vi "Estimator.vi"(0 "target_covariance":dbl[][](array[numeric]), 5 "nontarget_covariance":dbl[][](array[numeric]), 7 "u(t=1, 2, ...6)_target":dbl[][](array[numeric]), 9 "u(t=1, 2, ...6)_nontarget":dbl[][](array[numeric]), 11 "alk":dbl[][](array[numeric])) -> (4 "L_k(t)":ext[][](array[numeric]), 6 "H_lk":ext[][][](array[numeric]))   [LabVIEW 2013]
uses:
  <vilib>/Analysis/baseanly.llb/Real A x B.vi
  <vilib>/Analysis/Matrix/Numeric/Conversions/Array To Matrix - RA.vi
  <vilib>/Analysis/Matrix/Numeric/Conversions/Matrix To Array - RM.vi
  <vilib>/Analysis/Matrix/NI_Matrix.lvlib
  <vilib>/Analysis/NI_AALBase.lvlib
panel:
  in  "Tab Control":enum32{"ALPHA", "BETA", "L_K, H_KL"}(tab)
  out "pi":dbl[](array[numeric])
  out "u(1)_target":dbl[](array[numeric])
  out "u(1)_nontarget":dbl[](array[numeric])
  out "alpha_k(t)":ext[][](array[numeric])
  out "beta(t)":ext[][](array[numeric])
  out "P(u)":ext
  # "INPUT"
  # "INITIALIZATION"
  # "OUTPUT"
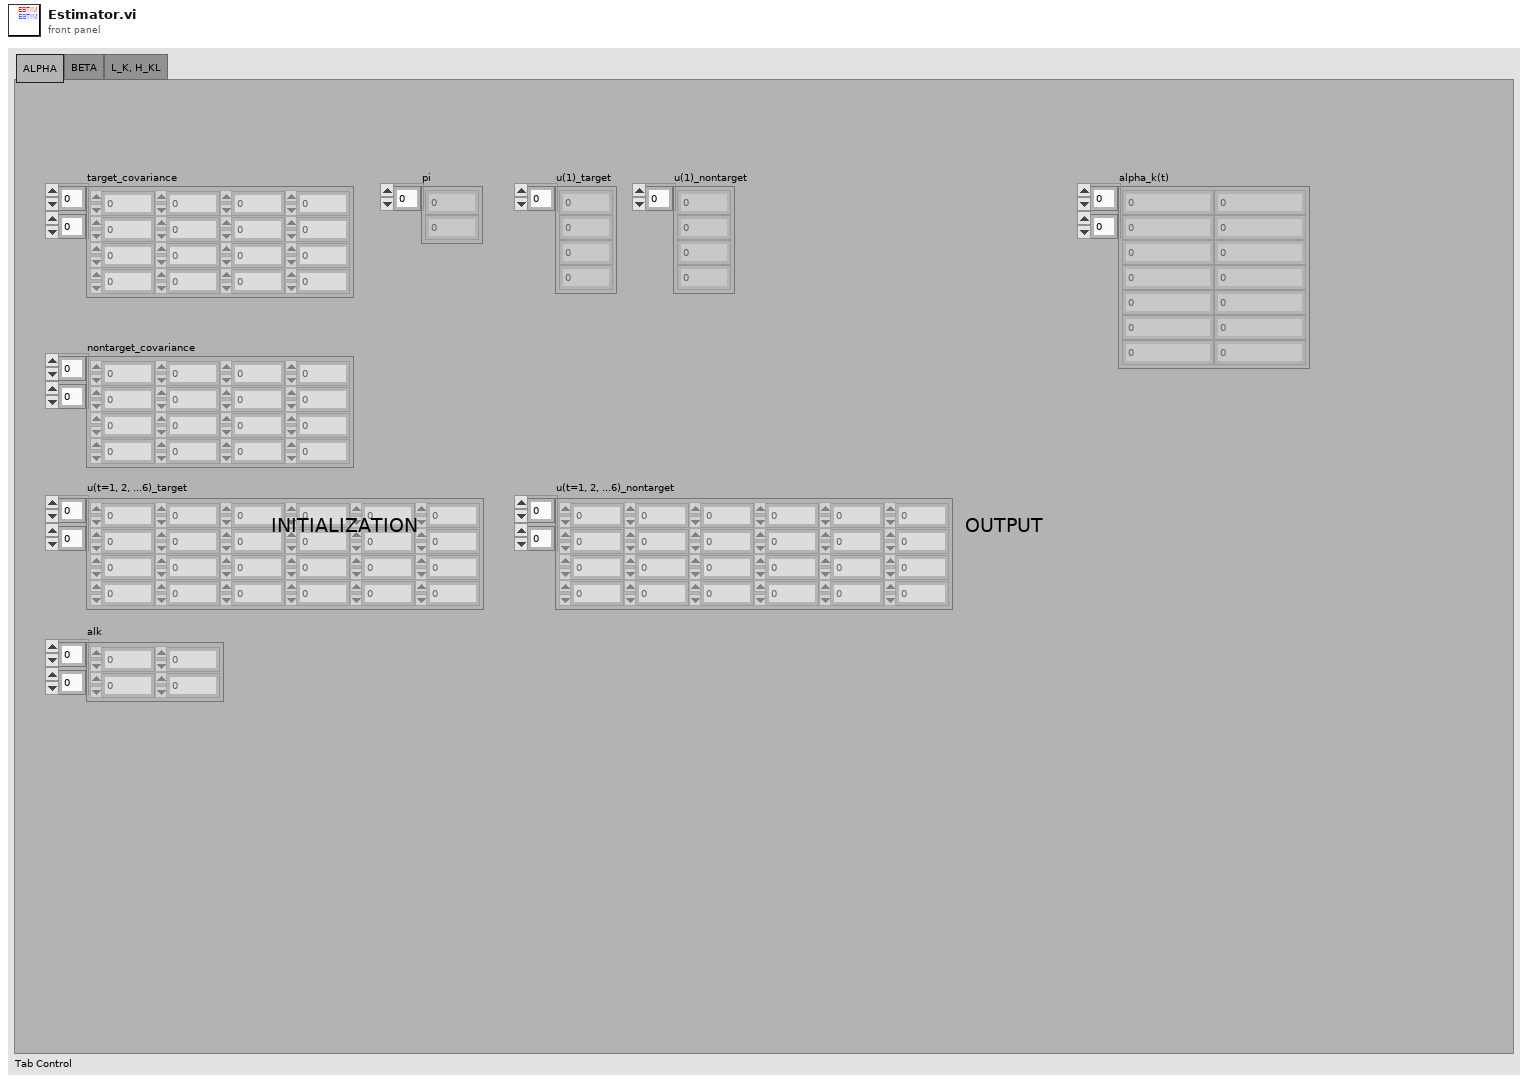
[diagram p1: front panel]
types:
  T1 = typedef "NI_Matrix.lvlib/RealMatrix.ctl" = dbl[][]
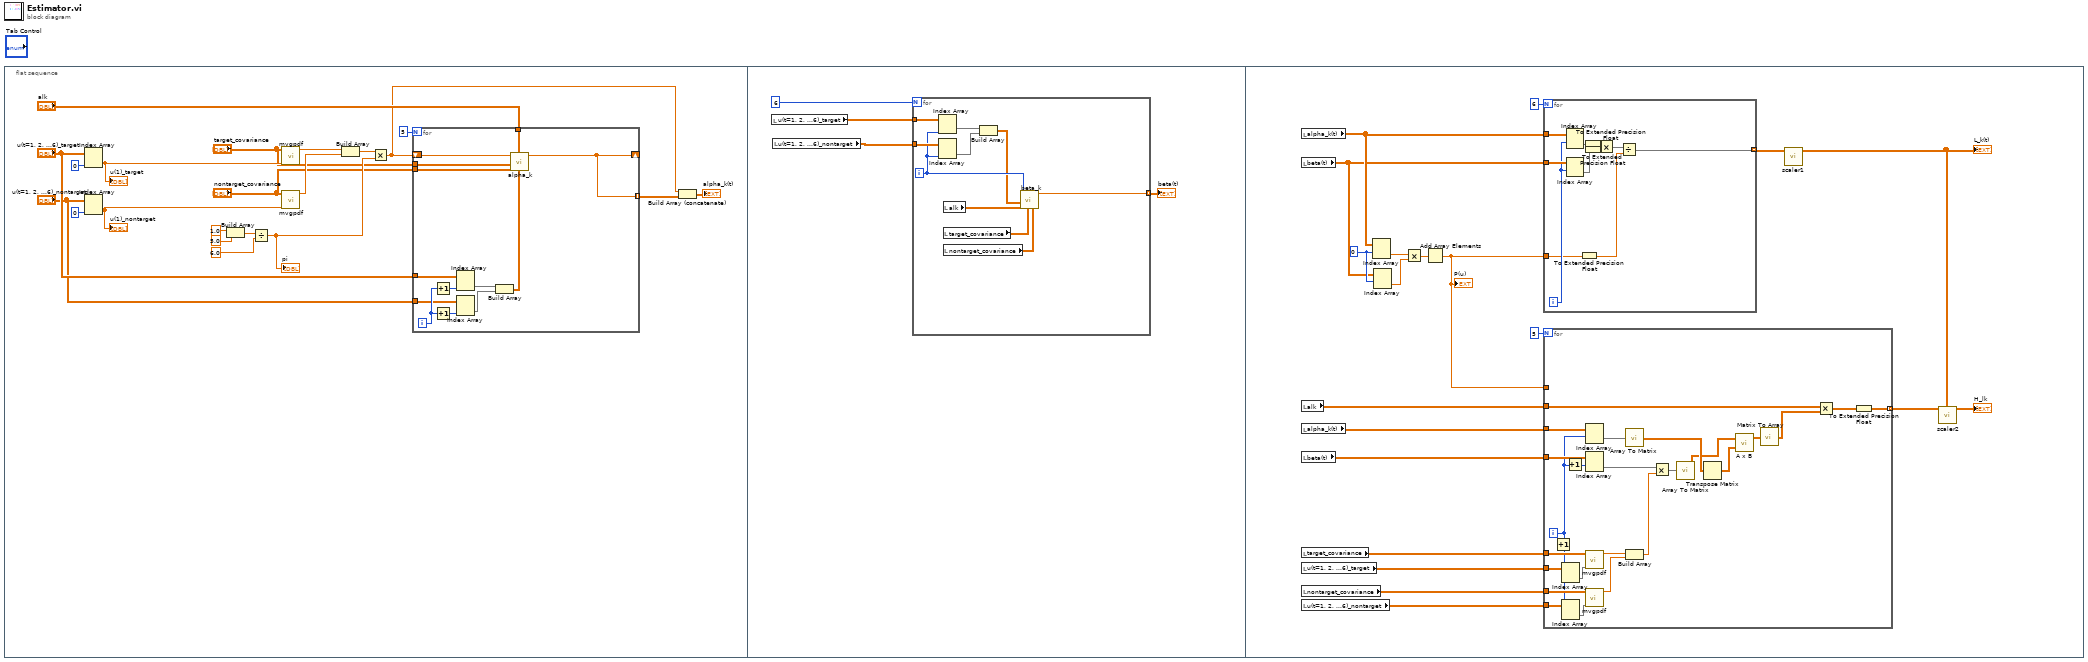
[diagram p0: block diagram]
diagram:
  n1 = flat-sequence {
    frame #0 {
      n2 = Index Array(array="u(t=1, 2, ...6)_target", index (col)=0 ("disabled index (col)")) -> (element=w16:dbl[])  [unwired: 1 in]
      "u(1)_target" <- w16
      n3 = Index Array(array="u(t=1, 2, ...6)_nontarget", index (col)=0 ("disabled index (col)")) -> (element=w7:dbl[])  [unwired: 1 in]
      "u(1)_nontarget" <- w7
      n4 = Build Array(1.0 ("element"), 5.0 ("element")) -> (w18:dbl[])
      n5 = Divide(x=w18, y=6.0) -> (x/y=w12:dbl[])
      "pi" <- w12
      n6 = call "mvgpdf.vi"("input_ERP(normalized)"=w16, "covariance"="target_covariance") -> ("Gaussian_prob"=w15:ext)  [unwired: 9 in]
      n7 = call "mvgpdf.vi"("input_ERP(normalized)"=w7, "covariance"="nontarget_covariance") -> ("Gaussian_prob"=w14:ext)  [unwired: 9 in]
      n8 = Build Array(w15, w14) -> (w13:ext[])
      n9 = Multiply(x=w13, y=w12) -> (x*y=w2:ext[])
      n10 = for {
        N: 5 -> [_]
        tunnel: "alk" -> [w34]
        tunnel: "target_covariance" -> [w32]
        tunnel: "nontarget_covariance" -> [w31]
        shift-right: [w22] -> _
        shift-left: w2 -> [w33]
        tunnel: "u(t=1, 2, ...6)_target" -> [w30]
        tunnel: "u(t=1, 2, ...6)_nontarget" -> [w26]
        tunnel: [w22] -> w3 mode=indexing
        i -> [w27]
        n11 = Increment(x=w27) -> (x+1=w29:i32)
        n12 = Increment(x=w27) -> (x+1=w28:i32)
        n13 = Index Array(array=w30, index (col)=w29) -> (element=w25:dbl[])  [unwired: 1 in]
        n14 = Index Array(array=w26, index (col)=w28) -> (element=w24:dbl[])  [unwired: 1 in]
        n15 = Build Array(w25, w24) -> (w23:dbl[][])
        n16 = call "alpha_k.vi"("u(t)"=w23, "alk"=w34, "nontarget_covariance"=w31, "target_covariance"=w32, "alpha(t-1)"=w33) -> ("alpha(t)"=w22:ext[])  [unwired: 6 in]
      }
      n17 = Build Array (concatenate)(w2, w3) -> (→"alpha_k(t)":ext[][])
    }
    frame #1 {
      n18 = local read "u(t=1, 2, ...6)_target"() -> (w37:dbl[][])
      n19 = local read "u(t=1, 2, ...6)_nontarget"() -> (w36:dbl[][])
      n20 = for {
        N: 6 -> [_]
        tunnel: w37 -> [w45]
        tunnel: w36 -> [w44]
        tunnel: [w39] -> w35 mode=indexing
        i -> [w43]
        n21 = Index Array(array=w45, index (col)=w43) -> (element=w42:dbl[])  [unwired: 1 in]
        n22 = Index Array(array=w44, index (col)=w43) -> (element=w41:dbl[])  [unwired: 1 in]
        n23 = local read "alk"() -> (w48:dbl[][])
        n24 = local read "target_covariance"() -> (w47:dbl[][])
        n25 = local read "nontarget_covariance"() -> (w46:dbl[][])
        n26 = Build Array(w42, w41) -> (w40:dbl[][])
        n27 = call "beta_k.vi"("covariance_nontarget"=w46, "covariance_target"=w47, "akl"=w48, "u(t+1) = current average"=w40, "T"=w43) -> ("beta(t)"=w39:ext[])  [unwired: 6 in]
      }
      "beta(t)" <- w35
    }
    frame #2 {
      w68 = 0 ("index (row)")
      n28 = local read "alpha_k(t)"() -> (w63:ext[][])
      n29 = local read "beta(t)"() -> (w62:ext[][])
      n30 = local read "alk"() -> (w55:dbl[][])
      n31 = local read "alpha_k(t)"() -> (w54:ext[][])
      n32 = local read "beta(t)"() -> (w53:ext[][])
      n33 = local read "target_covariance"() -> (w52:dbl[][])
      n34 = local read "u(t=1, 2, ...6)_target"() -> (w51:dbl[][])
      n35 = local read "nontarget_covariance"() -> (w50:dbl[][])
      n36 = local read "u(t=1, 2, ...6)_nontarget"() -> (w49:dbl[][])
      n37 = Index Array(array=w63, index (row)=w68) -> (element=w67:ext[])  [unwired: 1 in]
      n38 = Index Array(array=w62, index (row)=w68) -> (element=w66:ext[])  [unwired: 1 in]
      n39 = Multiply(x=w67, y=w66) -> (x*y=w65:ext[])
      n40 = Add Array Elements(numeric array=w65) -> (sum=w59:ext)
      "P(u)" <- w59
      n41 = for {
        N: 6 -> [_]
        tunnel: w63 -> [w104]
        tunnel: w62 -> [w103]
        tunnel: w59 -> [w98]
        tunnel: [w97] -> w61 mode=indexing
        i -> [w102]
        n42 = Index Array(array=w104, index (row)=w102) -> (element=w101:ext[])  [unwired: 1 in]
        n43 = Index Array(array=w103, index (row)=w102) -> (element=w100:ext[])  [unwired: 1 in]
        n44 = To Extended Precision Float(1:w98) -> (0:w94:ext)
        n45 = To Extended Precision Float(1:w101) -> (0:w96:ext[])
        n46 = To Extended Precision Float(1:w100) -> (0:w95:ext[])
        n47 = Multiply(x=w96, y=w95) -> (x*y=w99:ext[])
        n48 = Divide(x=w99, y=w94) -> (x/y=w97:ext[])
      }
      n49 = for {
        N: 5 -> [_]
        tunnel: w59 -> [_]
        tunnel: w54 -> [w93]
        tunnel: w53 -> [w92]
        tunnel: w55 -> [w73]
        tunnel: w52 -> [w90]
        tunnel: w50 -> [w89]
        tunnel: w51 -> [w87]
        tunnel: w49 -> [w84]
        tunnel: [w71] -> w58 mode=indexing
        i -> [w85]
        n50 = Increment(x=w85) -> (x+1=w83:i32)
        n51 = Index Array(array=w87, index (col)=w83) -> (element=w88:dbl[])  [unwired: 1 in]
        n52 = Index Array(array=w84, index (col)=w83) -> (element=w86:dbl[])  [unwired: 1 in]
        n53 = Increment(x=w85) -> (x+1=w91:i32)
        n54 = Index Array(array=w93, index (row)=w85) -> (element=w77:ext[])  [unwired: 1 in]
        n55 = Index Array(array=w92, index (row)=w91) -> (element=w80:ext[])  [unwired: 1 in]
        n56 = call "mvgpdf.vi"("input_ERP(normalized)"=w88, "covariance"=w90) -> ("Gaussian_prob"=w82:ext)  [unwired: 9 in]
        n57 = call "mvgpdf.vi"("input_ERP(normalized)"=w86, "covariance"=w89) -> ("Gaussian_prob"=w81:ext)  [unwired: 9 in]
        n58 = call-poly <vilib>:"Array To Matrix.vi"("Real 1D Array"=w77) -> ("Real Matrix (Column Vector)"=w70:T1)
        n59 = Build Array(w82, w81) -> (w79:ext[])
        n60 = Multiply(x=w80, y=w79) -> (x*y=w78:ext[])
        n61 = call-poly <vilib>:"Array To Matrix.vi"("Real 1D Array"=w78) -> ("Real Matrix (Column Vector)"=w69:T1)
        n62 = Transpose Matrix(1:w70) -> (0:w76:T1)
        n63 = call-poly <vilib>:"A x B.vi"("B"=w76, "A"=w69) -> ("A x B"=w75:T1)  [unwired: 1 out]
        n64 = call-poly <vilib>:"Matrix To Array.vi"("Real Matrix"=w75) -> ("Real 2D Array"=w72:dbl[][])
        n65 = Multiply(x=w73, y=w72) -> (x*y=w74:dbl[][])
        n66 = To Extended Precision Float(1:w74) -> (0:w71:ext[][])
      }
      n67 = call "scaler1.vi"("L_k(t)"=w61) -> ("L_k(t)"=w56:ext[][])  [unwired: 10 in]
      "L_k(t)" <- w56
      n68 = call "scaler2.vi"("L_k(t)"=w56, "H_lk"=w58) -> ("H_lk"=→"H_lk":ext[][][])  [unwired: 9 in]
    }
  }
